vi "Vision Processing.vi"(4 "error in (no error)":errorcluster, 7 "Image Size":T1=enum."320x240") -> ()   [LabVIEW 2013]
doc: "This VI runs in parallel to other tasks. It gets images from the camera, processes them for color or shape and use that information to affect robot behavior."
uses:
  <vilib>/Rock Robotics/WPI/Camera/WPI_CameraImageSize.ctl
  <vilib>/Rock Robotics/WPI/Camera/WPI_CameraWhite Balance Values.ctl
  <vilib>/Rock Robotics/WPI/Camera/WPI_CameraExposure Values.ctl
  <vilib>/Rock Robotics/WPI/Camera/WPI_CameraFrameRate.ctl
  Robot Global Data.vi
  <vilib>/vision/NI_Vision_Development_Module.lvlib
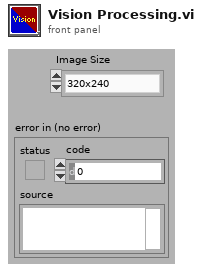
[diagram p1: front panel]
types:
  T1 = typedef "WPI_CameraImageSize.ctl" = enum16{"640x480", "320x240", "160x120"}
  T2 = typedef "WPI_CameraFrameRate.ctl" = u32
  T3 = typedef "WPI_CameraExposure Values.ctl" = enum16{"Auto", "Flicker-free 50 Hz", "Flicker-free 60 Hz", "Hold current"}
  T4 = typedef "WPI_CameraWhite Balance Values.ctl" = enum16{"Auto", "Fixed indoor", "Fixed outdoor 1", "Fixed outdoor 2", "Fixed fluorescent 1", "Fixed fluorescent 2", "Hold current"}
  T5 = typedef "Image Type" = u32
  T6 = typedef "WPI_CameraDevRef.ctl" = cluster{"Camera Address":string, "CameraStatus":errorcluster, "Acquire Image Notifier":refnum<notifier>}
  T7 = typedef "IMAQ Image.ctl" = refnum<image>
  T8 = typedef "Color (U64)" = cluster{"Plane 3 (Blue)":u16, "Plane 2 (Green)":u16, "Plane 1 (Red)":u16, "Plane 4 (alpha)":u16}
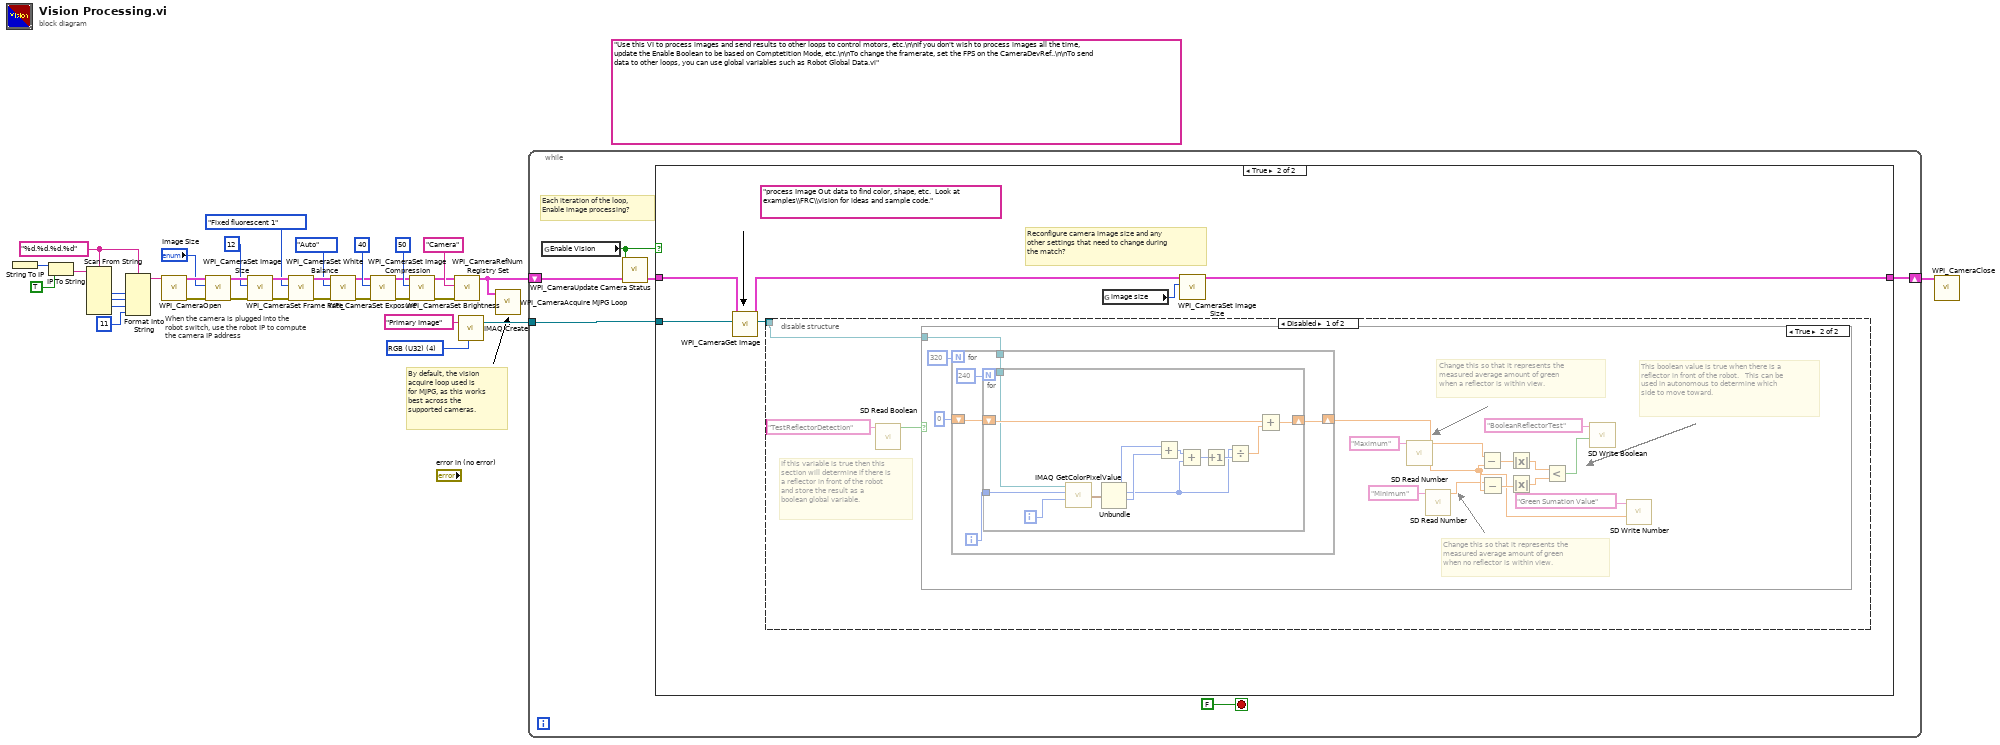
[diagram p0: block diagram]
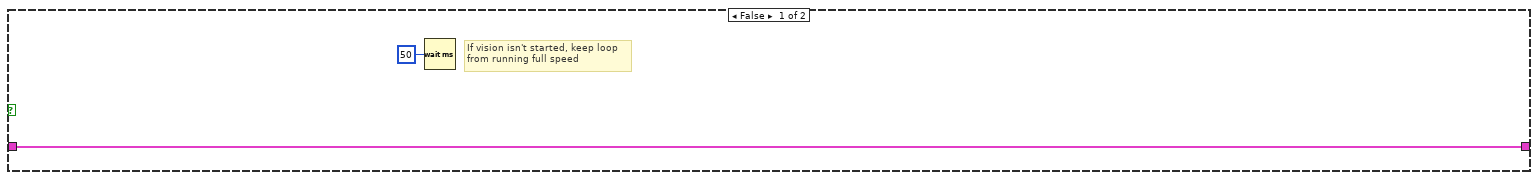
[diagram p2: hidden frame]
diagram:
  w5 = "%d.%d.%d.%d" ("format string")
  (unwired) "Use this VI to process images and send results to other loops to control motors, etc.\n\nIf you don't wish to process images all the time, update the Enable Boolean to be based on Comptetition Mode, etc.\n\nTo change the framerate, set the FPS on the CameraDevRef..\n\nTo send data to other loops, you can use global variables such as Robot Global Data.vi"
  w35 = T5 4 items=["Grayscale (U8)", "Grayscale (I16)", "Grayscale (SGL)", "Complex (CSG)", "RGB (U32)", "HSL (U32)", "RGB (U64)"] ("Image Type")
  # "When the camera is plugged into the\nrobot switch, use the robot IP to compute\nthe camera IP address"
  # "By default, the vision\nacquire loop used is\nfor MJPG, as this works\nbest across the\nsupported cameras."
  n1 = String To IP() -> (0:w12:u32)  [unwired: 1 in]
  n2 = IP To String(1:TRUE ("dot notation? (F)"), 2:w12) -> (0:w10:string)
  n3 = Scan From String(format string=w5, input string=w10) -> (output 1=w9:i32, output 2=w8:i32, output 3=w7:i32)  [unwired: 7 in, 3 out]
  n4 = Format Into String(format string=w5, w9, w8, w7, 11 ("Compression")) -> (resulting string=w4:string)  [unwired: 2 in, 1 out]
  n5 = call <vilib>:"WPI_CameraOpen.vi"("Camera Address"=w4) -> ("error out"=w23:errorcluster, "CameraDevRef"=w24:T6)  [unwired: 1 in, 8 out]
  n6 = call <vilib>:"WPI_CameraSet Image Size.vi"("error in (no error)"=w23, "Image Size"="Image Size", "CameraDevRef"=w24) -> ("error out"=w22:errorcluster, "CameraDevRef Out"=w25:T6)  [unwired: 7 out]
  n7 = call <vilib>:"WPI_CameraSet Frame Rate.vi"("error in (no error)"=w22, "Frame Rate (fps)"=T2 12, "CameraDevRef"=w25) -> ("error out"=w21:errorcluster, "CameraDevRef Out"=w27:T6)  [unwired: 7 out]
  n8 = call <vilib>:"WPI_CameraSet White Balance.vi"("error in (no error)"=w21, "White Balance"=WPI_CameraWhite_Balance_Values."Fixed fluorescent 1", "CameraDevRef"=w27) -> ("error out"=w20:errorcluster, "CameraDevRef Out"=w26:T6)  [unwired: 7 out]
  n9 = call <vilib>:"WPI_CameraSet Exposure.vi"("error in (no error)"=w20, "Exposure"=WPI_CameraExposure_Values."Auto", "CameraDevRef"=w26) -> ("error out"=w19:errorcluster, "CameraDevRef Out"=w29:T6)  [unwired: 7 out]
  n10 = call <vilib>:"WPI_CameraSet Image Compression.vi"("error in (no error)"=w19, "Compression"=40, "CameraDevRef"=w29) -> ("error out"=w18:errorcluster, "CameraDevRef Out"=w28:T6)  [unwired: 7 out]
  n11 = call <vilib>:"WPI_CameraSet Brightness.vi"("error in (no error)"=w18, "Brightness"=50, "CameraDevRef"=w28) -> ("error out"=w16:errorcluster, "CameraDevRef Out"=w17:T6)  [unwired: 7 out]
  n12 = call <vilib>:"WPI_CameraRefNum Registry Set.vi"("error in (no error)"=w16, "refnum name"="Camera", "CameraDevRef"=w17) -> ("CameraDevRef"=w3:T6)  [unwired: 8 out]
  n13 = call "IMAQ Create"("Image Name"="Primary Image", "Image Type"=w35) -> ("New Image"=w33:T7)  [unwired: 2 in, 2 out]
  n14 = call <vilib>:"WPI_CameraAcquire MJPG Loop.vi"("CameraDevRef"=w3) -> ()  [unwired: 11 in]
  n15 = while {
    shift-right: [w40] -> w1
    shift-left: w3 -> [w38]
    tunnel: w33 -> [w39]
    stop <- FALSE stop-if-true
    # "Each iteration of the loop,\nEnable image processing?"
    n16 = global read "Robot Global Data.vi" "Enable Vision"() -> (w36:bool)
    n17 = call <vilib>:"WPI_CameraUpdate Camera Status.vi"("CameraDevRef In"=w38, "Enable Vision"=w36) -> ("CameraDevRef Out"=w37:T6)  [unwired: 3 in]
    n18 = case shown="True" w36 {
      tunnel: w39 -> [_ w48]
      tunnel: [w43 w49] -> w40
      tunnel: w37 -> [w43 w46]
      frame False {
        # "If vision isn't started, keep loop\nfrom running full speed"
        n19 = Wait (ms)(milliseconds to wait=u32 50) -> ()  [unwired: 1 out]
      }
      frame True {
        (unwired) "process Image Out data to find color, shape, etc.  Look at examples\\FRC\\vision for ideas and sample code."
        # "Reconfigure camera image size and any\nother settings that need to change during\nthe match?"
        n20 = call <vilib>:"WPI_CameraGet Image.vi"("Image"=w48, "CameraDevRef"=w46) -> ("Image Out"=w44:T7, "CameraDevRef Out"=w45:T6)  [unwired: 1 in, 7 out]
        n21 = disable-structure shown="Disabled" {
          disable-tunnel: w44 -> [w52 _]
          frame Disabled {
            # "If this variable is true then this section will determine if there is a reflector in front of the robot and store the result as a boolean global variable."
            n22 = call <vilib>:"SD Read Boolean.vi"("Name"="TestReflectorDetection") -> ("Boolean"=w51:bool)  [unwired: 8 in, 2 out]
            n23 = case shown="True" w51 {
              tunnel: w52 -> [_ w61]
              frame False {
              }
              frame True {
                # "This boolean value is true when there is a reflector in front of the robot.   This can be used in autonomous to determine which side to move toward."
                # "Change this so that it represents the measured average amount of green\nwhen a reflector is within view."
                # "Change this so that it represents the measured average amount of green\nwhen no reflector is within view."
                n24 = for {
                  N: 320 -> [_]
                  shift-right: [w69] -> w60
                  shift-left: 0 -> [w70]
                  tunnel: w61 -> [w68]
                  i -> [w71]
                  n25 = for {
                    N: 240 -> [_]
                    tunnel: w71 -> [w84]
                    shift-right: [w81] -> w69
                    shift-left: w70 -> [w82]
                    tunnel: w68 -> [w80]
                    i -> [w85]
                    n26 = call "IMAQ GetColorPixelValue"("Y Coordinate"=w85, "X Coordinate"=w84, "Image"=w80) -> ("Pixel Value (U64)"=w83:T8)  [unwired: 1 in, 2 out]
                    n27 = Unbundle(w83) -> ("Plane 3 (Blue)"=w76:u16, "Plane 2 (Green)"=w73:u16, "Plane 1 (Red)"=w77:u16)  [unwired: 1 out]
                    n28 = Add(x=w76, y=w77) -> (x+y=w74:u16)
                    n29 = Add(x=w74, y=w73) -> (x+y=w75:u16)
                    n30 = Increment(x=w75) -> (x+1=w78:u16)
                    n31 = Divide(x=w73, y=w78) -> (x/y=w79:dbl)
                    n32 = Add(x=w82, y=w79) -> (x+y=w81:dbl)
                  }
                }
                n33 = call <vilib>:"SD Read Number.vi"("Name"="Maximum") -> ("Numeric"=w56:dbl)  [unwired: 8 in, 2 out]
                n34 = call <vilib>:"SD Read Number.vi"("Name"="Minimum") -> ("Numeric"=w53:dbl)  [unwired: 8 in, 2 out]
                n35 = Subtract(x=w56, y=w60) -> (x-y=w65:dbl)
                n36 = Subtract(x=w53, y=w60) -> (x-y=w63:dbl)
                n37 = Absolute Value(x=w65) -> (abs(x)=w64:dbl)
                n38 = Absolute Value(x=w63) -> (abs(x)=w62:dbl)
                n39 = Less?(x=w64, y=w62) -> (x < y?=w58:bool)
                n40 = call <vilib>:"SD Write Boolean.vi"("Boolean"=w58, "Name"="BooleanReflectorTest") -> ()  [unwired: 8 in, 2 out]
                n41 = call <vilib>:"SD Write Number.vi"("Numeric"=w60, "Name"="Green Sumation Value") -> ()  [unwired: 8 in, 2 out]
              }
            }
          }
          frame Enabled {
          }
        }
        n42 = global read "Robot Global Data.vi" "image size"() -> (w47:T1)
        n43 = call <vilib>:"WPI_CameraSet Image Size.vi"("Image Size"=w47, "CameraDevRef"=w45) -> ("CameraDevRef Out"=w49:T6)  [unwired: 1 in, 8 out]
      }
    }
  }
  n44 = call <vilib>:"WPI_CameraClose.vi"("CameraDevRef"=w1) -> ()  [unwired: 1 in, 10 out]
